vi "ief_get_axis_following_error.vi"(3 "error in (no error)":errorcluster, 4 "Axis Number":u16=1 min=1 max=16, 5 "Tagprefix in":refnum<k21>) -> (0 "error out (no error)":errorcluster, 1 "Axis Following Error":dbl format="%.2f", 2 "Tagprefix out":refnum<k21>)   [LabVIEW 2015, in "IEF Werner.lvlib"]
doc: "The VI returns the present axis following error of the chosen axis.\n\nAxis Number Range:\n01, 10 hex\n1, 16 dec"
uses:
  IEF Werner.lvlib
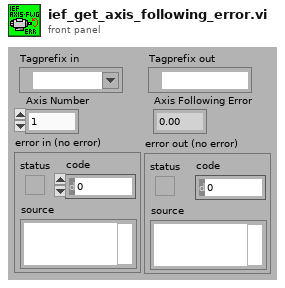
[diagram p1: front panel]
types:
  T1 = typedef "Semaphore RefNum" = refnum<k1>
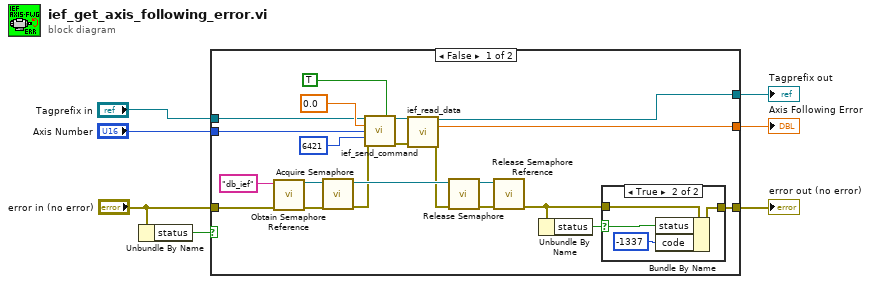
[diagram p0: block diagram]
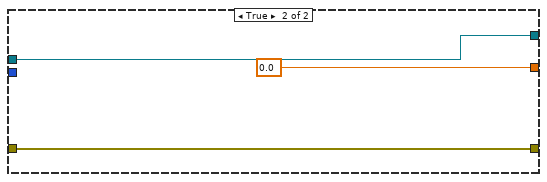
[diagram p3: hidden frame]
diagram:
  n1 = Unbundle By Name("error in (no error)") -> ("status"=w4:bool)
  n2 = case shown="False" w4 {
    tunnel: "Axis Number" -> [w26 _]
    tunnel: "error in (no error)" -> [w17 w36]
    tunnel: [w24 w36] -> w6
    tunnel: [w11 sgl 0.0 ("value real 32")] -> w3
    tunnel: "Tagprefix in" -> [w10 w35]
    tunnel: [w8 w35] -> w1
    frame False {
      n3 = call <vilib>:"Obtain Semaphore Reference.vi"("error in (no error)"=w17, "name (unnamed)"="db_ief") -> ("error out"=w21:errorcluster, "semaphore"=w22:T1)  [unwired: 3 in, 1 out]
      n4 = call <vilib>:"Acquire Semaphore.vi"("error in (no error)"=w21, "semaphore"=w22) -> ("error out"=w16:errorcluster, "semaphore out"=w20:T1)  [unwired: 3 in, 1 out]
      n5 = call "ief_send_command.vi"("Tagprefix in"=w10, "Command datum of type real"=TRUE, "Command datum"=sgl 0.0, "Command parameter"=w26, "Command code"=u16 6421, "error in (no error)"=w16) -> ("Tagprefix out"=w9:refnum<k21>, "error out (no error)"=w25:errorcluster)  [unwired: 4 in, 4 out]
      n6 = call "ief_read_data.vi"("Tagprefix in"=w9, "error in (no error)"=w25) -> ("Tagprefix out"=w8:refnum<k21>, "value real 32"=w11:sgl, "error out (no error)"=w15:errorcluster)  [unwired: 7 in, 4 out]
      n7 = call <vilib>:"Release Semaphore.vi"("error in (no error)"=w15, "semaphore"=w20) -> ("error out"=w19:errorcluster, "semaphore out"=w18:T1)  [unwired: 4 in]
      n8 = call <vilib>:"Release Semaphore Reference.vi"("error in (no error)"=w19, "semaphore"=w18) -> ("error out"=w14:errorcluster)  [unwired: 8 in, 1 out]
      n9 = Unbundle By Name(w14) -> ("status"=w12:bool)
      n10 = case shown="True" w12 {
        selector: w12 -> [_ w30]
        tunnel: [w29 w32] -> w24
        tunnel: w14 -> [w29 w33]
        frame False {
        }
        frame True {
          n11 = Bundle By Name(cluster=w33, "status"=w30, "code"=-1337) -> (w32:errorcluster)
        }
      }
    }
    frame True {
    }
  }
  "error out (no error)" <- w6
  "Axis Following Error" <- w3
  "Tagprefix out" <- w1
